vi "Launch TCP Loop.vi"(7 "Secure":bool, 8 "error in (no error)":errorcluster, 9 "Server URI":refnum<class "URI.lvclass">, 10 "TCP":refnum<k5>, 11 "Server in":refnum<class "Server.lvclass">) -> (0 "error out":errorcluster, 3 "Server out":refnum<class "Server.lvclass">)   [LabVIEW 2020, in "HTTP Server.lvlib" / "Server.lvclass"]
uses:
  Server.lvclass
  Server.lvclass/Server.ctl
  TCP Loop Async.vi
  lv-uri/URI/URI/URI.lvclass
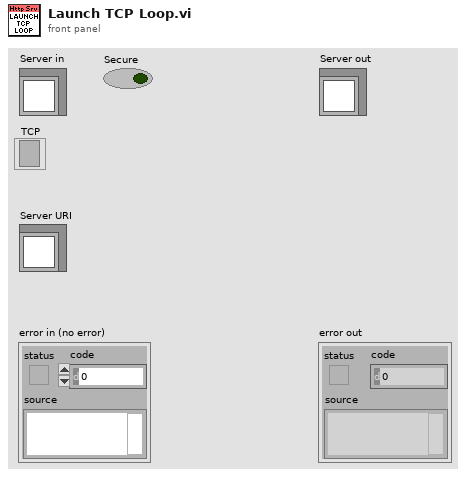
[diagram p1: front panel]
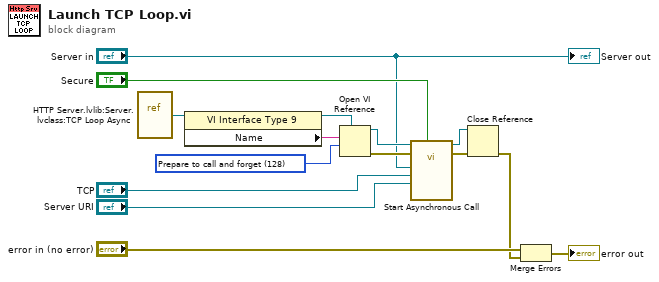
[diagram p0: block diagram]
diagram:
  w9 = 128 items=["Record modifications"=1, "Open templates for editing"=2, "Prompt user to save"=4, "Prepare for reentrant run"=8, "Prompt to find missing subVIs"=16, "Hide loading dialog box"=32, "Enable simultaneous calls"=64, "Prepare to call and forget"=128, "Simultaneous call and forget"=192, "Prepare to call and collect"=256, "Simultaneous call and collect"=320]
  n1 = vi-ref "HTTP Server.lvlib:Server.lvclass:TCP Loop Async.vi"() -> (w7:refnum<vi>)
  n2 = property class="VI Interface Type 9"(reference=w7) -> (reference out=w10:refnum<vi>, "Name"=w8:string)  [unwired: 1 in, 1 out]
  n3 = Open VI Reference(type specifier VI Refnum (for type only)=w10, vi path=w8, options=w9) -> (vi reference=w12:refnum<vi>, error out=w11:errorcluster)  [unwired: 3 in]
  n4 = call-by-ref "Start Asynchronous Call"(reference=w12, error in=w11, "Secure"="Secure", "Client URI"="Server URI", "TCP"="TCP", "Server in"="Server in") -> (reference out=w14:refnum<vi>, error out=w13:errorcluster)  [unwired: 8 in]
  n5 = Close Reference(reference=w14, error in (no error)=w13) -> (error out=w2:errorcluster)
  n6 = Merge Errors("error in (no error)", w2) -> (→"error out":errorcluster)
  "Server out" <- "Server in"
